vi "Auto Catapult.vi"(9 "Shoot":i32, 10 "Shoot Mode ID":i32) -> (3 "Finished?":bool)   [LabVIEW 2015]
uses:
  Common Code/Catapult/Catapult Manual Commands.ctl
  Common Code/Change Detect Boolean.vi
  Robot Global Data.vi
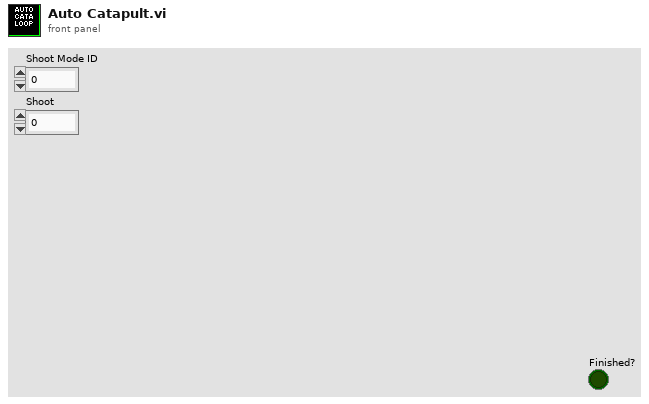
[diagram p1: front panel]
types:
  T1 = typedef "Catapult Manual Commands.ctl" = enum16{"Ready", "Release ", "Shoot"}
  T2 = typedef "Catapult Command Cluster.ctl" = cluster{"Auto Commands":T3, "Mode":T4, "Override IR":bool, "Shoot Mode":T5, "Shoot?":bool, "Manual Commands":T1, "Ball Loaded?":bool}
  T3 = typedef "Catapult Auto Commands.ctl" = enum16{"Idle", "Warmup", "Shoot"}
  T4 = typedef "Shoot Modes Enum.ctl" = enum16{"Manual", "Auto"}
  T5 = typedef "Shoot Mode.ctl" = enum16{"Outer", "Batter"}
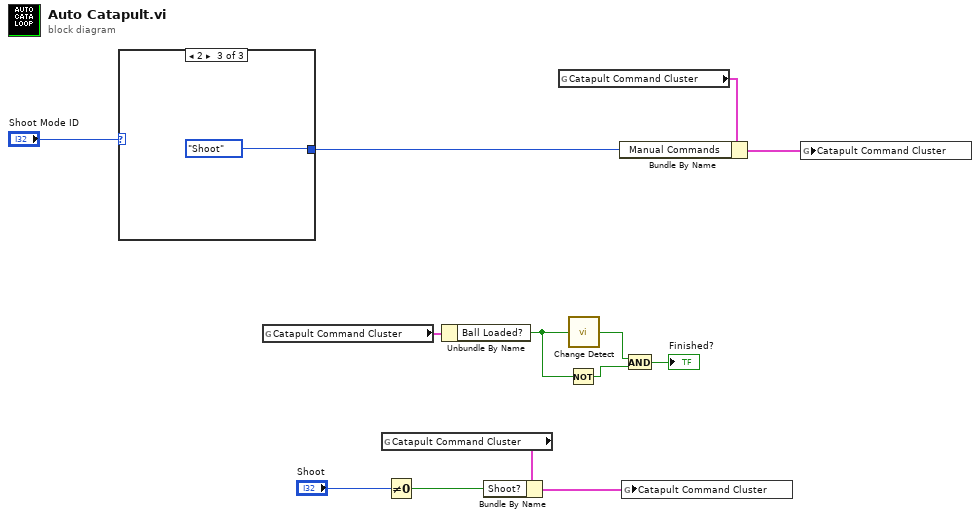
[diagram p0: block diagram]
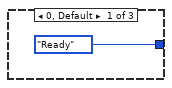
[diagram p2: hidden frame]
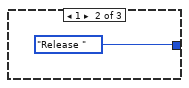
[diagram p3: hidden frame]
diagram:
  n1 = case shown="2" "Shoot Mode ID" {
    tunnel: [Catapult_Manual_Commands."Ready" ("Manual Commands") Catapult_Manual_Commands."Release " ("Manual Commands") Catapult_Manual_Commands."Shoot" ("Manual Commands")] -> w6
    frame 0, Default {
    }
    frame 1 {
    }
    frame 2 {
    }
  }
  n2 = global read "Robot Global Data.vi" "Catapult Command Cluster"() -> (w1:T2)
  n3 = global read "Robot Global Data.vi" "Catapult Command Cluster"() -> (w13:T2)
  n4 = Not Equal To 0?(x="Shoot") -> (x != 0?=w9:bool)
  n5 = Unbundle By Name(w1) -> ("Ball Loaded?"=w5:bool)
  n6 = Bundle By Name(cluster=w13, "Shoot?"=w9) -> (w12:T2)
  n7 = global read "Robot Global Data.vi" "Catapult Command Cluster"() -> (w8:T2)
  n8 = Not(x=w5) -> (.not. x?=w4:bool)
  n9 = call-poly "Change Detect.vi"("In"=w5) -> ("Changed?"=w3:bool)
  n10 = Bundle By Name(cluster=w8, "Manual Commands"=w6) -> (w7:T2)
  n11 = global write "Robot Global Data.vi" "Catapult Command Cluster"(w12) -> ()
  n12 = And(x=w3, y=w4) -> (x .and. y?=→"Finished?":bool)
  n13 = global write "Robot Global Data.vi" "Catapult Command Cluster"(w7) -> ()
